vi "VendingMachine.vi"() -> ()   [LabVIEW 2020]
uses:
  VendingMachineController.ctl
panel:
  out "Estado":T1=enum."Fin"
  in  "$10 2":dbl=5.0 format="%#_13g"
  in  "$5 2":dbl=5.0 format="%#_13g"
  out "Dinero Total":dbl
  in  "$10":bool
  in  "Comenzar":bool
  out "Alertas":string
  out "Costo de Seleccion":dbl
  in  "Comprar":bool
  out "Dinero recibido":dbl
  out "$5":dbl
  out "$10":dbl
  out "$1":dbl
  out "Diez  pesos":dbl caption="10  pesos"
  out "Cinco pesos":dbl caption="5 pesos"
  out "Un peso":dbl caption="1 peso"
  in  "Salir":bool
  in  "$5":bool
  in  "$1":bool
  out "Fanta":dbl
  out "Ameyal":dbl
  out "Fresca":dbl
  in  "Fanta":bool
  in  "Fresca":bool
  in  "Ameyal":bool
  # "Inventario"
  # "Cambio"
  # "Precio"
  # "Dinero por \nDenominacion"
  # "$8"
  # "$10"
  # "$12"
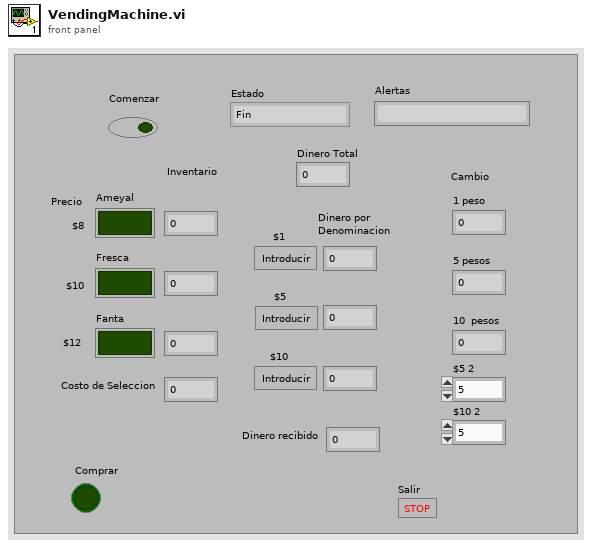
[diagram p1: front panel]
types:
  T1 = typedef "VendingMachineController.ctl" = enum16{"Inicio", "Comparar", "Cambio", "Fin"}
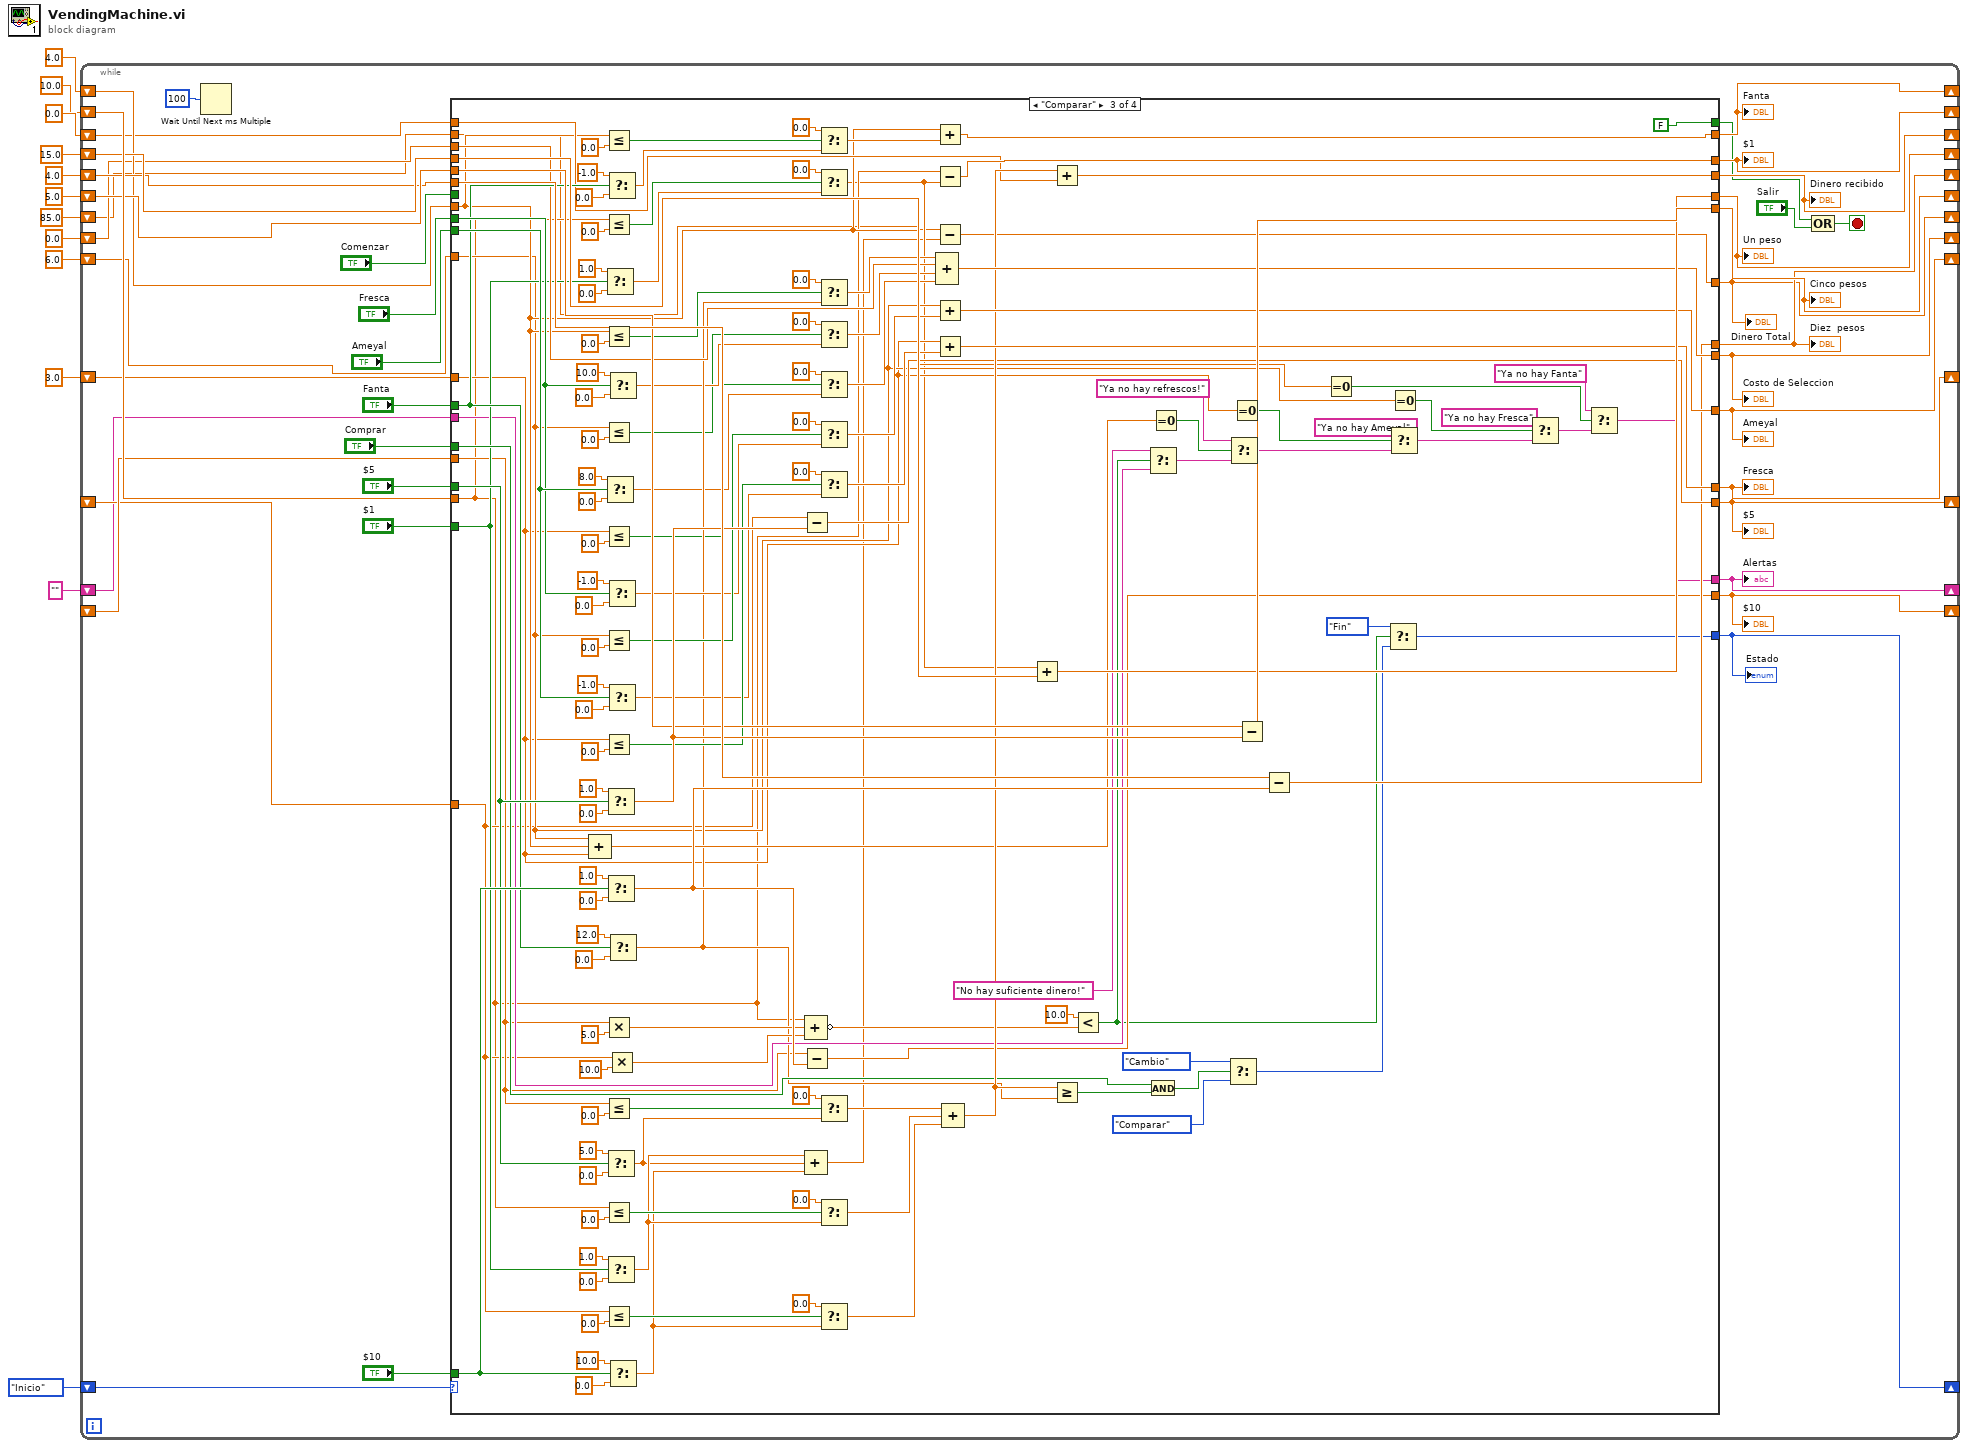
[diagram p0: block diagram]
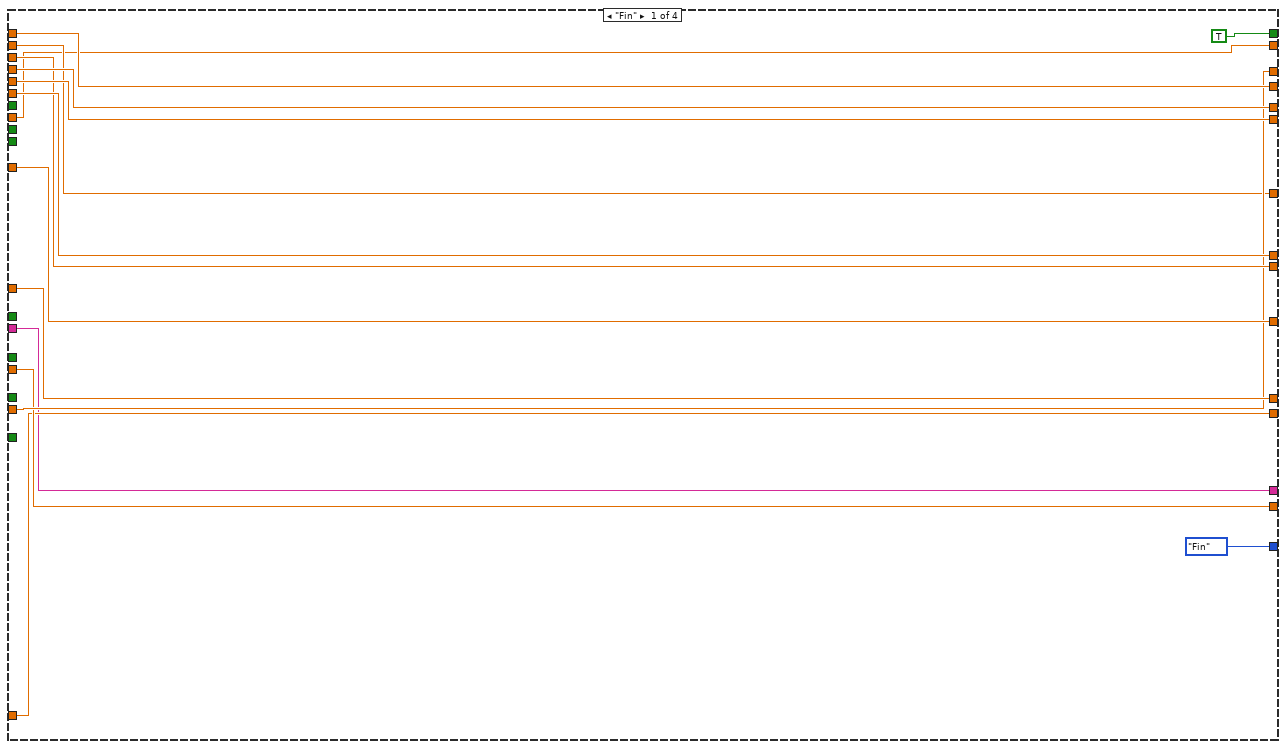
[diagram p2: hidden frame]
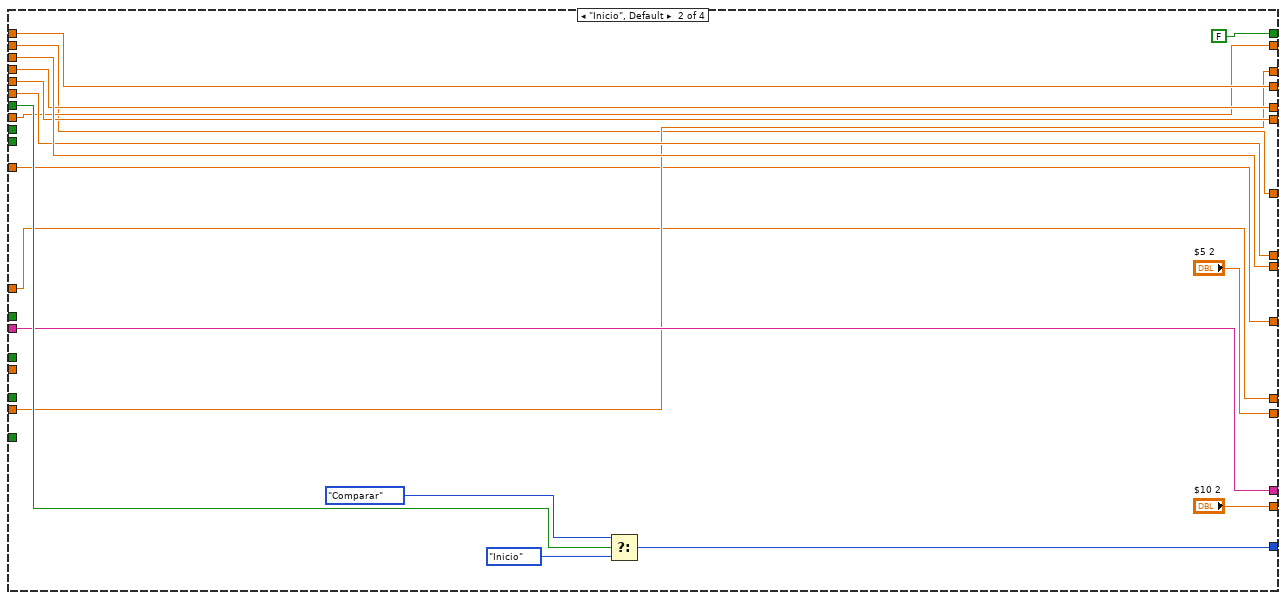
[diagram p3: hidden frame]
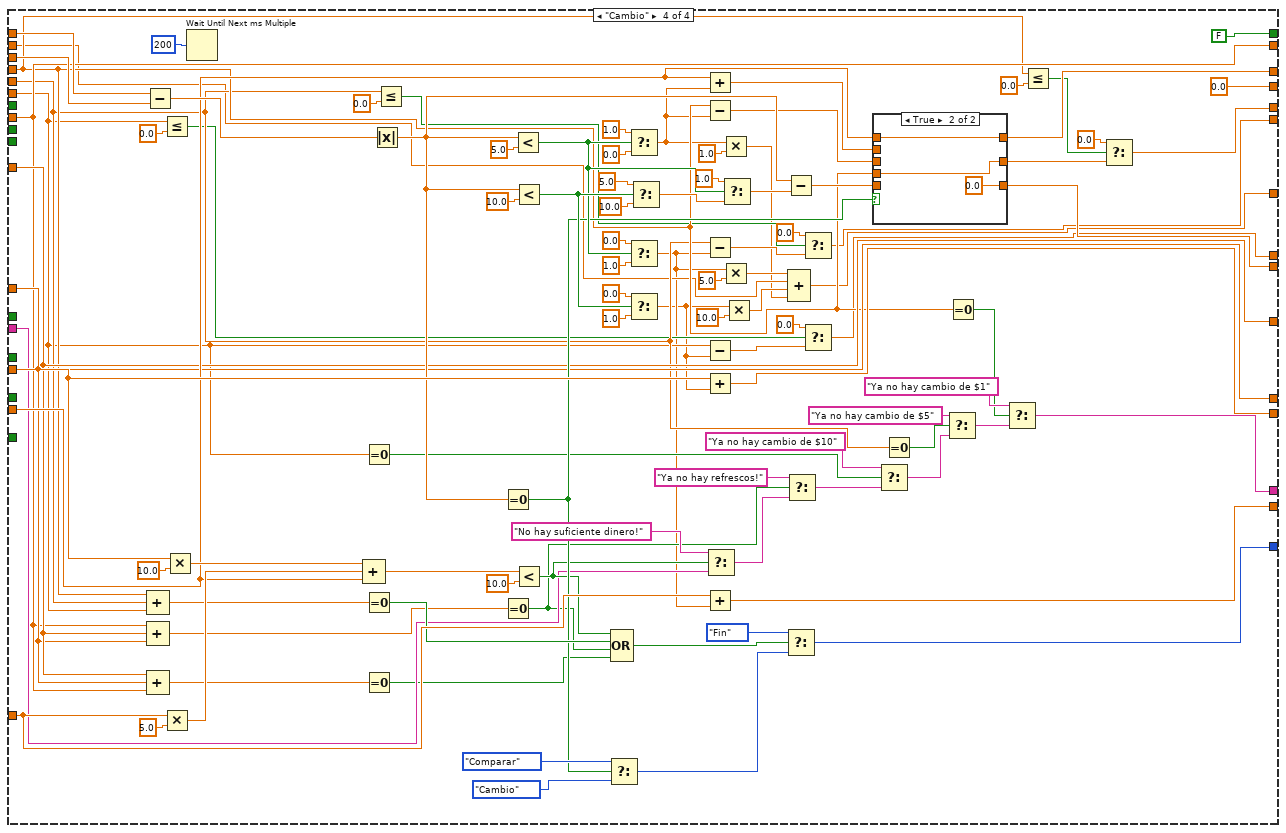
[diagram p4: hidden frame]
diagram:
  n1 = while {
    shift-right: [w51] -> _
    shift-left: 10.0 ("$1") -> [w52]
    shift-right: [w18] -> _
    shift-left: _ -> [w49]
    shift-right: [w19] -> _
    shift-left: _ -> [w50]
    shift-right: [w22] -> _
    shift-left: 15.0 ("$10") -> [w43]
    shift-right: [w40] -> _
    shift-left: 5.0 ("$10") -> [w42]
    shift-right: [w39] -> _
    shift-left: 4.0 ("$10") -> [w41]
    shift-right: [w33] -> _
    shift-left: 3.0 ("$10") -> [w38]
    shift-right: [w34] -> _
    shift-left: 6.0 ("$10") -> [w37]
    shift-right: [w35] -> _
    shift-left: 4.0 ("$10") -> [w36]
    shift-right: [w13] -> _
    shift-left: VendingMachineController."Inicio" -> [w28]
    shift-right: [w32] -> _
    shift-left: 0.0 ("Total") -> [w31]
    shift-right: [w29] -> _
    shift-left: 0.0 ("Total") -> [w30]
    shift-right: [w21] -> _
    shift-left: "" -> [w20]
    shift-right: [w15] -> _
    shift-left: 85.0 ("$10") -> [w14]
    stop <- w25 stop-if-true
    n2 = Wait Until Next ms Multiple(millisecond multiple=u32 100) -> ()  [unwired: 1 out]
    n3 = case shown="\"Comparar\"" w28 {
      tunnel: "Ameyal" -> [_ _ w197 _]
      tunnel: "Fresca" -> [_ _ w193 _]
      tunnel: "Fanta" -> [_ _ w189 _]
      tunnel: "$1" -> [_ _ w176 _]
      tunnel: "$5" -> [_ _ w208 _]
      tunnel: "$10" -> [_ _ w213 _]
      tunnel: [VendingMachineController."Fin" w85 w158 w301] -> w13
      tunnel: w52 -> [w58 w74 w95 w278]
      tunnel: [w58 w74 w200 w279] -> w51
      tunnel: w50 -> [w57 _ w99 w295]
      tunnel: w49 -> [w56 _ w98 w294]
      tunnel: [w57 "$10 2" w153 w306] -> w19
      tunnel: [w56 "$5 2" w175 w305] -> w18
      tunnel: [w61 w75 w198 w251] -> w22
      tunnel: w43 -> [w61 w75 w199 w249]
      tunnel: [w64 w76 w203 w245] -> w40
      tunnel: w42 -> [w64 w76 w204 w243]
      tunnel: [w62 w77 w174 w238] -> w39
      tunnel: w41 -> [w62 w77 w209 w237]
      tunnel: [w63 w73 w194 w261] -> w33
      tunnel: w38 -> [w63 w73 w112 w261]
      tunnel: [w65 w72 w190 w262] -> w34
      tunnel: w37 -> [w65 w72 w120 w262]
      tunnel: [w53 w71 w186 w260] -> w35
      tunnel: w36 -> [w53 w71 w128 w260]
      tunnel: [w60 w82 w183 0.0 ("Total")] -> w32
      tunnel: w31 -> [w60 w82 w179 w323]
      tunnel: w30 -> [w59 w81 w182 w322]
      tunnel: [w59 w81 w181 w283] -> w29
      tunnel: [TRUE FALSE FALSE FALSE] -> w26
      tunnel: "Comenzar" -> [_ w79 _ _]
      tunnel: "Comprar" -> [_ _ w178 _]
      tunnel: [w55 w78 w165 w269] -> w21
      tunnel: w20 -> [w55 w78 w154 w266]
      tunnel: [w54 w70 w86 w235] -> w15
      tunnel: w14 -> [w54 w70 w91 w236]
      frame "Fin" {
      }
      frame "Inicio", Default {
        n4 = Select(t=VendingMachineController."Comparar", s=w79, f=VendingMachineController."Inicio") -> (s? t:f=w85:T1)
      }
      frame "Comparar" {
        n5 = Compound Arithmetic op=ADD(w120, w128, w112) -> (w149:dbl)
        n6 = Less Or Equal?(x=w128, y=0.0) -> (x <= y?=w145:bool)
        n7 = Less Or Equal?(x=w95, y=0.0) -> (x <= y?=w97:bool)
        n8 = Less Or Equal?(x=w128, y=0.0) -> (x <= y?=w130:bool)
        n9 = Less Or Equal?(x=w120, y=0.0) -> (x <= y?=w121:bool)
        n10 = Less Or Equal?(x=w112, y=0.0) -> (x <= y?=w117:bool)
        n11 = Less Or Equal?(x=w120, y=0.0) -> (x <= y?=w141:bool)
        n12 = Less Or Equal?(x=w112, y=0.0) -> (x <= y?=w135:bool)
        n13 = Multiply(x=w99, y=5.0) -> (x*y=w162:dbl)
        n14 = Less Or Equal?(x=w99, y=0.0) -> (x <= y?=w111:bool)
        n15 = Less Or Equal?(x=w95, y=0.0) -> (x <= y?=w108:bool)
        n16 = Less Or Equal?(x=w98, y=0.0) -> (x <= y?=w105:bool)
        n17 = Select(t=1.0, s=w176, f=0.0) -> (s? t:f=w93:dbl)
        n18 = Select(t=8.0, s=w197, f=0.0) -> (s? t:f=w115:dbl)
        n19 = Select(t=1.0, s=w208, f=0.0) -> (s? t:f=w205:dbl)
        n20 = Select(t=1.0, s=w213, f=0.0) -> (s? t:f=w210:dbl)
        n21 = Select(t=5.0, s=w208, f=0.0) -> (s? t:f=w89:dbl)
        n22 = Select(t=1.0, s=w176, f=0.0) -> (s? t:f=w90:dbl)
        n23 = Select(t=-1.0, s=w189, f=0.0) -> (s? t:f=w144:dbl)
        n24 = Select(t=-1.0, s=w193, f=0.0) -> (s? t:f=w138:dbl)
        n25 = Select(t=-1.0, s=w197, f=0.0) -> (s? t:f=w133:dbl)
        n26 = Multiply(x=w98, y=10.0) -> (x*y=w163:dbl)
        n27 = Select(t=10.0, s=w193, f=0.0) -> (s? t:f=w123:dbl)
        n28 = Select(t=12.0, s=w189, f=0.0) -> (s? t:f=w126:dbl)
        n29 = Select(t=10.0, s=w213, f=0.0) -> (s? t:f=w88:dbl)
        n30 = Subtract(x=w98, y=w205) -> (x-y=w175:dbl)
        n31 = Subtract(x=w99, y=w210) -> (x-y=w153:dbl)
        n32 = Compound Arithmetic op=ADD(w95, w162, w163) -> (invert w155:dbl)
        n33 = Compound Arithmetic op=ADD(w90, w89, w88) -> (w87:dbl)
        n34 = Select(t=0.0, s=w145, f=w144) -> (s? t:f=w143:dbl)
        n35 = Select(t=0.0, s=w97, f=w93) -> (s? t:f=w92:dbl)
        n36 = Select(t=0.0, s=w130, f=w126) -> (s? t:f=w125:dbl)
        n37 = Select(t=0.0, s=w121, f=w123) -> (s? t:f=w118:dbl)
        n38 = Select(t=0.0, s=w117, f=w115) -> (s? t:f=w113:dbl)
        n39 = Select(t=0.0, s=w141, f=w138) -> (s? t:f=w137:dbl)
        n40 = Select(t=0.0, s=w135, f=w133) -> (s? t:f=w132:dbl)
        n41 = Select(t=0.0, s=w111, f=w89) -> (s? t:f=w102:dbl)
        n42 = Select(t=0.0, s=w108, f=w90) -> (s? t:f=w101:dbl)
        n43 = Select(t=0.0, s=w105, f=w88) -> (s? t:f=w100:dbl)
        n44 = Add(x=w128, y=w143) -> (x+y=w186:dbl)
        n45 = Subtract(x=w95, y=w92) -> (x-y=w200:dbl)
        n46 = Subtract(x=w91, y=w87) -> (x-y=w86:dbl)
        n47 = Add(x=w120, y=w137) -> (x+y=w190:dbl)
        n48 = Add(x=w112, y=w132) -> (x+y=w194:dbl)
        n49 = Compound Arithmetic op=ADD(w125, w182, w118, w113) -> (w181:dbl)
        n50 = Compound Arithmetic op=ADD(w102, w101, w100) -> (w180:dbl)
        n51 = Add(x=w92, y=w199) -> (x+y=w198:dbl)
        n52 = Add(x=w180, y=w179) -> (x+y=w183:dbl)
        n53 = Greater Or Equal?(x=w180, y=w126) -> (x >= y?=w177:bool)
        n54 = Less?(x=10.0 ("y"), y=w155) -> (x < y?=w152:bool)
        n55 = Select(t="No hay suficiente dinero!", s=w152, f=w154) -> (s? t:f=w150:string)
        n56 = And(x=w178, y=w177) -> (x .and. y?=w185:bool)
        n57 = Equal To 0?(x=w149) -> (x = 0?=w148:bool)
        n58 = Select(t=VendingMachineController."Cambio", s=w185, f=VendingMachineController."Comparar") -> (s? t:f=w159:T1)
        n59 = Select(t="Ya no hay refrescos!", s=w148, f=w150) -> (s? t:f=w151:string)
        n60 = Equal To 0?(x=w112) -> (x = 0?=w166:bool)
        n61 = Subtract(x=w204, y=w205) -> (x-y=w203:dbl)
        n62 = Subtract(x=w209, y=w210) -> (x-y=w174:dbl)
        n63 = Equal To 0?(x=w128) -> (x = 0?=w167:bool)
        n64 = Select(t=VendingMachineController."Fin", s=w152, f=w159) -> (s? t:f=w158:T1)
        n65 = Select(t="Ya no hay Ameyal", s=w166, f=w151) -> (s? t:f=w172:string)
        n66 = Equal To 0?(x=w120) -> (x = 0?=w168:bool)
        n67 = Select(t="Ya no hay Fresca", s=w168, f=w172) -> (s? t:f=w171:string)
        n68 = Select(t="Ya no hay Fanta", s=w167, f=w171) -> (s? t:f=w165:string)
      }
      frame "Cambio" {
        n69 = Subtract(x=w323, y=w322) -> (x-y=w286:dbl)
        n70 = Compound Arithmetic op=ADD(w249, w243, w237) -> (w291:dbl)
        n71 = Compound Arithmetic op=ADD(w260, w262, w261) -> (w289:dbl)
        n72 = Compound Arithmetic op=ADD(w262, w261, w260) -> (w264:dbl)
        n73 = Less Or Equal?(x=w237, y=0.0) -> (x <= y?=w242:bool)
        n74 = Multiply(x=w294, y=5.0) -> (x*y=w296:dbl)
        n75 = Multiply(x=w295, y=10.0) -> (x*y=w298:dbl)
        n76 = Wait Until Next ms Multiple(millisecond multiple=u32 200) -> ()  [unwired: 1 out]
        n77 = Compound Arithmetic op=ADD(w298, w296, w278) -> (w293:dbl)
        n78 = Equal To 0?(x=w237) -> (x = 0?=w272:bool)
        n79 = Equal To 0?(x=w291) -> (x = 0?=w290:bool)
        n80 = Equal To 0?(x=w264) -> (x = 0?=w263:bool)
        n81 = Absolute Value(x=w286) -> (abs(x)=w285:dbl)
        n82 = Less Or Equal?(x=w243, y=0.0) -> (x <= y?=w247:bool)
        n83 = Equal To 0?(x=w285) -> (x = 0?=w284:bool)
        n84 = Equal To 0?(x=w289) -> (x = 0?=w256:bool)
        n85 = Less?(x=w285, y=5.0) -> (x < y?=w307:bool)
        n86 = Less?(x=w285, y=10.0) -> (x < y?=w314:bool)
        n87 = Less?(x=w293, y=10.0) -> (x < y?=w267:bool)
        n88 = Select(t=VendingMachineController."Comparar", s=w284, f=VendingMachineController."Cambio") -> (s? t:f=w302:T1)
        n89 = Compound Arithmetic op=OR(w267, w290, w256, w263) -> (w265:bool)
        n90 = Select(t=1.0, s=w307, f=0.0) -> (s? t:f=w228:dbl)
        n91 = Select(t=0.0, s=w307, f=1.0) -> (s? t:f=w234:dbl)
        n92 = Select(t=0.0, s=w314, f=1.0) -> (s? t:f=w231:dbl)
        n93 = Select(t=5.0, s=w314, f=10.0) -> (s? t:f=w318:dbl)
        n94 = Add(x=w278, y=w228) -> (x+y=w280:dbl)
        n95 = Subtract(x=w249, y=w228) -> (x-y=w281:dbl)
        n96 = Subtract(x=w243, y=w234) -> (x-y=w246:dbl)
        n97 = Subtract(x=w237, y=w231) -> (x-y=w239:dbl)
        n98 = Add(x=w295, y=w231) -> (x+y=w305:dbl)
        n99 = Add(x=w294, y=w234) -> (x+y=w306:dbl)
        n100 = Select(t="No hay suficiente dinero!", s=w267, f=w266) -> (s? t:f=w258:string)
        n101 = Multiply(x=w228, y=1.0) -> (x*y=w226:dbl)
        n102 = Multiply(x=w234, y=5.0) -> (x*y=w232:dbl)
        n103 = Select(t=1.0, s=w307, f=w318) -> (s? t:f=w315:dbl)
        n104 = Multiply(x=w231, y=10.0) -> (x*y=w229:dbl)
        n105 = Subtract(x=w285, y=w315) -> (x-y=w282:dbl)
        n106 = Select(t=VendingMachineController."Fin", s=w265, f=w302) -> (s? t:f=w301:T1)
        n107 = Select(t="Ya no hay refrescos!", s=w256, f=w258) -> (s? t:f=w259:string)
        n108 = Compound Arithmetic op=ADD(w232, w236, w229, w226) -> (w235:dbl)
        n109 = Select(t=0.0, s=w247, f=w246) -> (s? t:f=w245:dbl)
        n110 = Select(t=0.0, s=w242, f=w239) -> (s? t:f=w238:dbl)
        n111 = case shown="True" w284 {
          tunnel: [w326 0.0] -> w283
          tunnel: w282 -> [w326 _]
          tunnel: w281 -> [w325 _]
          tunnel: [w325 w327] -> w252
          tunnel: w280 -> [w324 _]
          tunnel: [w324 w328] -> w279
          tunnel: w278 -> [_ w328]
          tunnel: w249 -> [_ w327]
          frame False {
          }
          frame True {
          }
        }
        n112 = Select(t="Ya no hay cambio de $10", s=w272, f=w259) -> (s? t:f=w274:string)
        n113 = Equal To 0?(x=w243) -> (x = 0?=w270:bool)
        n114 = Select(t="Ya no hay cambio de $5", s=w270, f=w274) -> (s? t:f=w276:string)
        n115 = Equal To 0?(x=w249) -> (x = 0?=w271:bool)
        n116 = Select(t="Ya no hay cambio de $1", s=w271, f=w276) -> (s? t:f=w269:string)
        n117 = Less Or Equal?(x=w249, y=0.0) -> (x <= y?=w254:bool)
        n118 = Select(t=0.0, s=w254, f=w252) -> (s? t:f=w251:dbl)
      }
    }
    "$1" <- w51
    "$5" <- w18
    "$10" <- w19
    "Fresca" <- w33
    "Ameyal" <- w34
    "Fanta" <- w35
    "Cinco pesos" <- w40
    "Diez  pesos" <- w39
    "Dinero recibido" <- w32
    "Costo de Seleccion" <- w29
    "Un peso" <- w22
    "Alertas" <- w21
    "Dinero Total" <- w15
    "Estado" <- w13
    n119 = Compound Arithmetic op=OR(w26, "Salir") -> (w25:bool)
  }
